vi "clone.vi"(0 "reference":refnum<class "GeneralPathEdge.lvclass">, 5 "error in (no error)":errorcluster) -> (14 "reference out":refnum<class "GeneralPathEdge.lvclass">, 15 "clonedEdge":refnum<class "AbstractEdge.lvclass">, 19 "error out":errorcluster)   [LabVIEW 2014, in "GeneralPathEdge.lvclass"]
doc: "Clone"
uses:
  <resource>/Framework/Providers/Open_GDS/UML/GeneralPathEdge_class/GeneralPathEdge.lvclass
  <resource>/Framework/Providers/Open_GDS/UML/AbstractEdge_class/AbstractEdge.lvclass
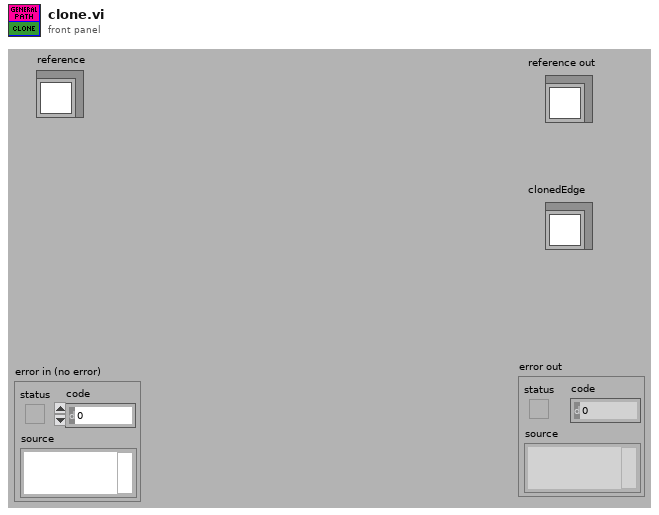
[diagram p1: front panel]
types:
  T1 = typedef "GeneralPathEdge.lvclass/ObjectAttributes.ctl" = cluster{"None":bool}
  T2 = typedef "AbstractEdge.lvclass/ObjectAttributes.ctl" = cluster{"start":refnum<class "AbstractNode.lvclass">, "end":refnum<class "AbstractNode.lvclass">}
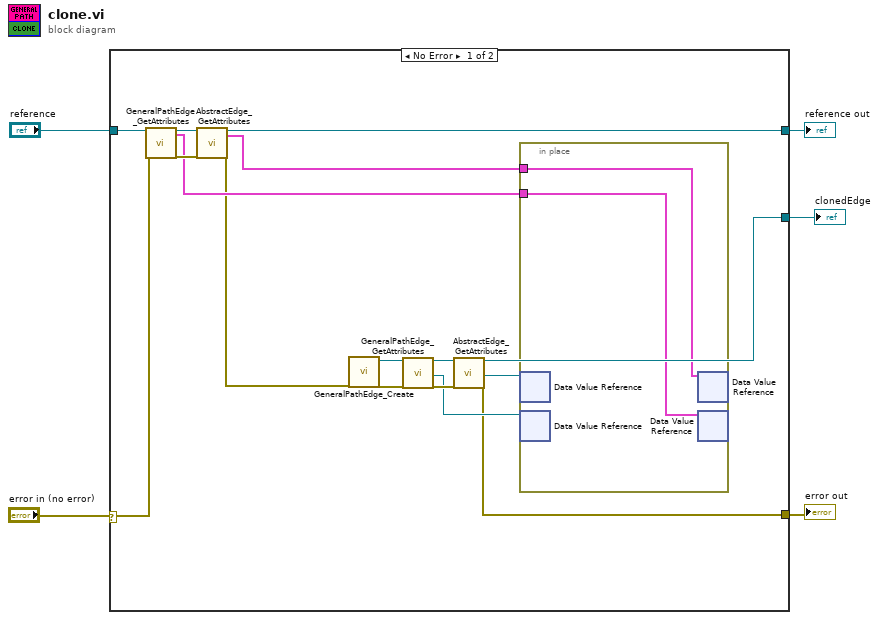
[diagram p0: block diagram]
diagram:
  n1 = case shown="No Error" "error in (no error)" {
    selector: "error in (no error)" -> [w9 w24]
    tunnel: "reference" -> [w14 w25]
    tunnel: [w8 w24] -> w4
    tunnel: [w12 w25] -> w3
    tunnel: [w7 _] -> w1
    frame No Error {
      n2 = call <resource>:"GeneralPathEdge_GetAttributes.vi"("reference in"=w14, "error in (no error)"=w9) -> ("reference out"=w13:refnum<class "GeneralPathEdge.lvclass">, "Data"=w18:T1, "error out"=w21:errorcluster)  [unwired: 14 in, 1 out]
      n3 = call <resource>:"AbstractEdge_GetAttributes.vi"("reference in"=w13, "error in (no error)"=w21) -> ("reference out"=w12:refnum<class "GeneralPathEdge.lvclass">, "Data"=w17:T2, "error out"=w10:errorcluster)  [unwired: 14 in, 1 out]
      n4 = call <resource>:"GeneralPathEdge_Create.vi"("error in (no error)"=w10) -> ("reference out"=w6:refnum<class "GeneralPathEdge.lvclass">, "error out"=w11:errorcluster)  [unwired: 17 in]
      n5 = call <resource>:"GeneralPathEdge_GetAttributes.vi"("reference in"=w6, "error in (no error)"=w11) -> ("reference out"=w19:refnum<class "GeneralPathEdge.lvclass">, "DataRef"=w15:refnum<data-value>, "error out"=w20:errorcluster)  [unwired: 14 in, 1 out]
      n6 = call <resource>:"AbstractEdge_GetAttributes.vi"("reference in"=w19, "error in (no error)"=w20) -> ("reference out"=w7:refnum<class "GeneralPathEdge.lvclass">, "DataRef"=w16:refnum<data-value>, "error out"=w8:errorcluster)  [unwired: 14 in, 1 out]
      n7 = in-place {
        in-place-border: w18 -> [w23]
        in-place-border: w17 -> [w22]
        n8 = in-place-dvr #1(w16) -> ()  [unwired: 2 out]
        n9 = in-place-dvr #2(w15) -> ()  [unwired: 2 out]
        n10 = in-place-dvr #1(w22) -> ()  [unwired: 2 out]
        n11 = in-place-dvr #2(w23) -> ()  [unwired: 2 out]
      }
    }
    frame Error {
    }
  }
  "reference out" <- w3
  "error out" <- w4
  "clonedEdge" <- w1
